vi "Read Value.vi"(8 "error in (no error)":errorcluster, 11 "Nested Value Update Msg in":refnum<class "Nested Value Update Msg.lvclass">) -> (0 "error out":errorcluster, 2 "Value":variant, 3 "Nested Value Update Msg out":refnum<class "Nested Value Update Msg.lvclass">)   [LabVIEW 2015, in "IViewable.lvlib" / "Nested Value Update Msg.lvclass"]
uses:
  Nested Value Update Msg.lvclass
  Nested Value Update Msg.lvclass/Nested Value Update Msg.ctl
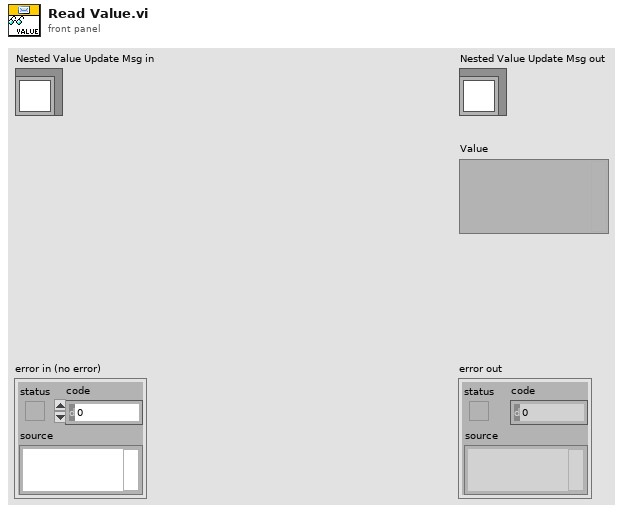
[diagram p1: front panel]
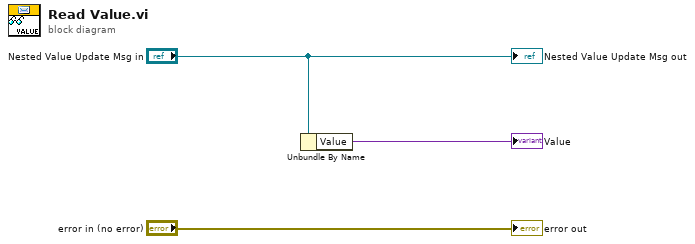
[diagram p0: block diagram]
diagram:
  n1 = Unbundle By Name("Nested Value Update Msg in") -> ("Value"=→"Value":variant)
  "error out" <- "error in (no error)"
  "Nested Value Update Msg out" <- "Nested Value Update Msg in"
